vi "VIPM_Find File Group Name.vi"(8 "error in (no error)":errorcluster, 11 "Refnum in":T1) -> (0 "error out":errorcluster, 2 "File Group Name":string, 3 "Refnum out":T1)   [LabVIEW 2019, in "Project.Dependencies Finder.lvlib" / "Dependency Source_VIPM.lvclass"]
doc: "Find the file group with most files and get the group name. Only groups that have a supported 'Target Dir' can be found.\nSupported 'Target Dir's:\n<application>"
uses:
  Dependency Source_VIPM.lvclass
  <vilib>/Utility/config.llb/Config Data RefNum.ctl
  <vilib>/Utility/config.llb/NI_LVConfig.lvlib
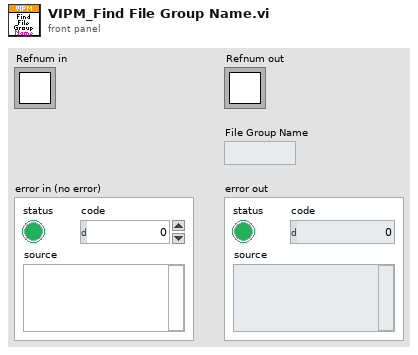
[diagram p1: front panel]
types:
  T1 = typedef "NI_LVConfig.lvlib/Config Data RefNum.ctl" = refnum<k1>
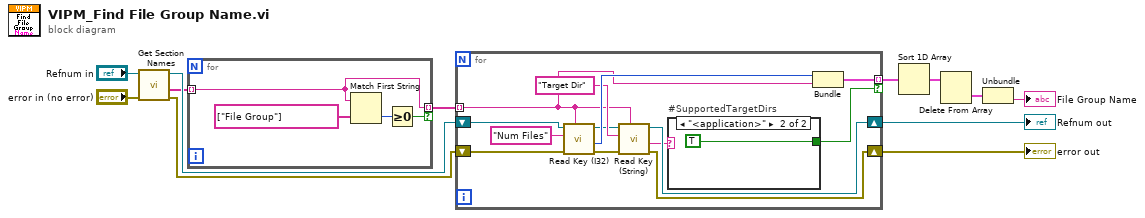
[diagram p0: block diagram]
diagram:
  n1 = call <vilib>:"Get Section Names.vi"("error in (no error)"="error in (no error)", "refnum"="Refnum in") -> ("error out"=w6:errorcluster, "section names"=w2:string[], "refnum out"=w4:T1)  [unwired: 7 in]
  n2 = for {
    tunnel: w2 -> [w14] mode=indexing
    tunnel: [w14] -> w3 mode=indexing if=w13
    n3 = Match First String(2:string[] ["File Group"], 3:w14) -> (0:w15:i32)  [unwired: 1 out]
    n4 = Greater Or Equal To 0?(x=w15) -> (x >= 0?=w13:bool)
  }
  n5 = for {
    tunnel: w3 -> [w23] mode=indexing
    shift-right: [w21] -> w10
    shift-left: w4 -> [w28]
    shift-right: [w19] -> w11
    shift-left: w6 -> [w27]
    tunnel: [w25] -> w7 mode=indexing if=w17
    n6 = call <vilib>:"Read Key (I32).vi"("section"=w23, "error in (no error)"=w27, "key"="Num Files", "refnum"=w28) -> ("error out"=w20:errorcluster, "value"=w26:i32, "refnum out"=w22:T1)  [unwired: 4 in, 1 out]
    n7 = call <vilib>:"Read Key (String).vi"("section"=w23, "error in (no error)"=w20, "key"="Target Dir", "refnum"=w22) -> ("error out"=w19:errorcluster, "value"=w18:string, "refnum out"=w21:T1)  [unwired: 4 in, 1 out]
    n8 = case "#SupportedTargetDirs" shown="\"<application>\"" w18 {
      tunnel: [_ TRUE] -> w17
      frame Default {
      }
      frame "<application>" {
      }
    }
    n9 = Bundle("value"=w26, "String"=w23) -> (w25:cluster{"value":i32, "String":string})  [unwired: 1 in]
  }
  "error out" <- w11
  "Refnum out" <- w10
  n10 = Sort 1D Array(array=w7) -> (sorted array=w8:cluster{"value":i32, "String":string}[])
  n11 = Delete From Array(array=w8) -> (deleted portion=w9:cluster{"value":i32, "String":string})  [unwired: 2 in, 1 out]
  n12 = Unbundle(w9) -> ("String"=→"File Group Name":string)  [unwired: 1 out]
